vi "Sub_Build_Fixed_Header.vi"(6 "Remaining Length":u32, 7 "Retain":T1, 8 "error in (no error)":errorcluster, 9 "QoS":T2, 10 "DUP":T3, 11 "MessageType":T4=enum."CONNECT") -> (0 "error out":errorcluster, 3 "Fixed Header":u8[](array[numeric]) format="%x")   [LabVIEW 2018, in "MQTT_Functions.lvlib"]
uses:
  MQTT_Functions.lvlib
  Controls/MessageType.ctl
  Controls/DUP_Flag.ctl
  Controls/QoS.ctl
  Controls/Retain_Flag.ctl
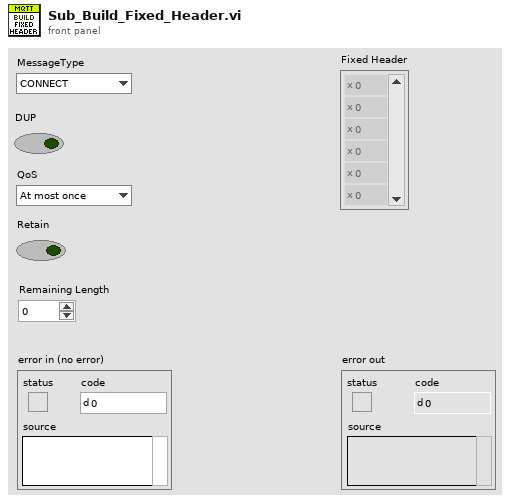
[diagram p1: front panel]
types:
  T1 = typedef "MQTT_Functions.lvlib/Retain_Flag.ctl" = bool
  T2 = typedef "MQTT_Functions.lvlib/QoS.ctl" = enum8{"At most once", "At least once", "Exactly once", "Reserved"}
  T3 = typedef "MQTT_Functions.lvlib/DUP_Flag.ctl" = bool
  T4 = typedef "MQTT_Functions.lvlib/MessageType.ctl" = enum32{"Reserved", "CONNECT", "CONNACK", "PUBLISH", "PUBACK", "PUBREC", "PUBREL", "PUBCOMP", "SUBSCRIBE", "SUBACK", "UNSUBSCRIBE", "UNSUBACK", "PINGREQ", "PINGRESP", "DISCONNECT", "Reserved2"}
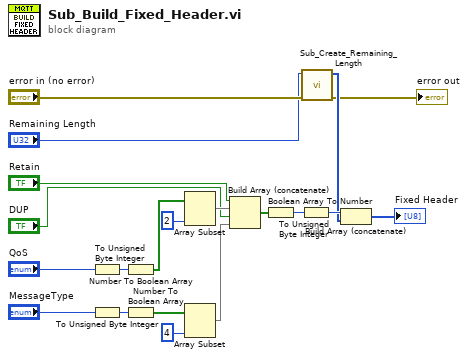
[diagram p0: block diagram]
diagram:
  n1 = To Unsigned Byte Integer(number="QoS") -> (unsigned 8bit integer=w18:u8)
  n2 = To Unsigned Byte Integer(number="MessageType") -> (unsigned 8bit integer=w19:u8)
  n3 = Number To Boolean Array(number=w18) -> (Boolean array=w14:bool[])
  n4 = Number To Boolean Array(number=w19) -> (Boolean array=w16:bool[])
  n5 = Array Subset(array=w14, length=2) -> (w3:bool[])  [unwired: 1 in]
  n6 = Array Subset(array=w16, length=4) -> (w1:bool[])  [unwired: 1 in]
  n7 = Build Array (concatenate)("Retain", w3, "DUP", w1) -> (w12:T3[])
  n8 = Boolean Array To Number(Boolean array=w12) -> (number=w11:u32)
  n9 = To Unsigned Byte Integer(number=w11) -> (unsigned 8bit integer=w10:u8)
  n10 = call "Sub_Create_Remaining_Length.vi"("error in (no error)"="error in (no error)", "X"="Remaining Length") -> ("error out"=→"error out":errorcluster, "bytes"=w9:u8[])  [unwired: 8 in]
  n11 = Build Array (concatenate)(w10, w9) -> (→"Fixed Header":u8[])
